vi "Test UI.vi"() -> ()   [LabVIEW 2014, in "UI Reference tests.lvlib"]
uses:
  UI Reference tests.lvlib
panel:
  out "String ind":string
  in  "String ctl":string
  out "Boolean ind":bool
  in  "Boolean ctl":bool
  out "Double ind":dbl
  in  "Double ctl":dbl
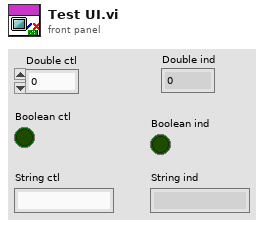
[diagram p1: front panel]
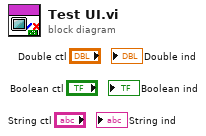
[diagram p0: block diagram]
diagram:
